vi "Threshold and Subsample Image.vi"(6 "Subsample":i32=1, 9 "Threshold":u8, 10 "Direction to keep":enum16{"Above", "Below"}(ring), 11 "Image Pixels (U8)":u8[][](array[numeric])) -> (1 "Cross Threshold Points":cluster{"X":i32, "Y":i32}[](array[cluster]), 3 "Image Pixels (U8) out":u8[][](array[numeric]))   [LabVIEW 2013]
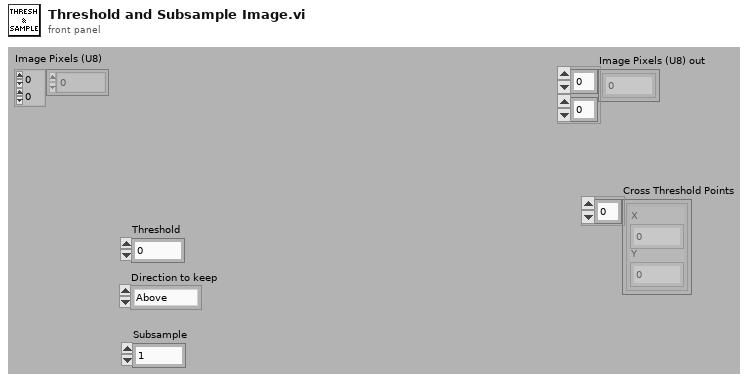
[diagram p1: front panel]
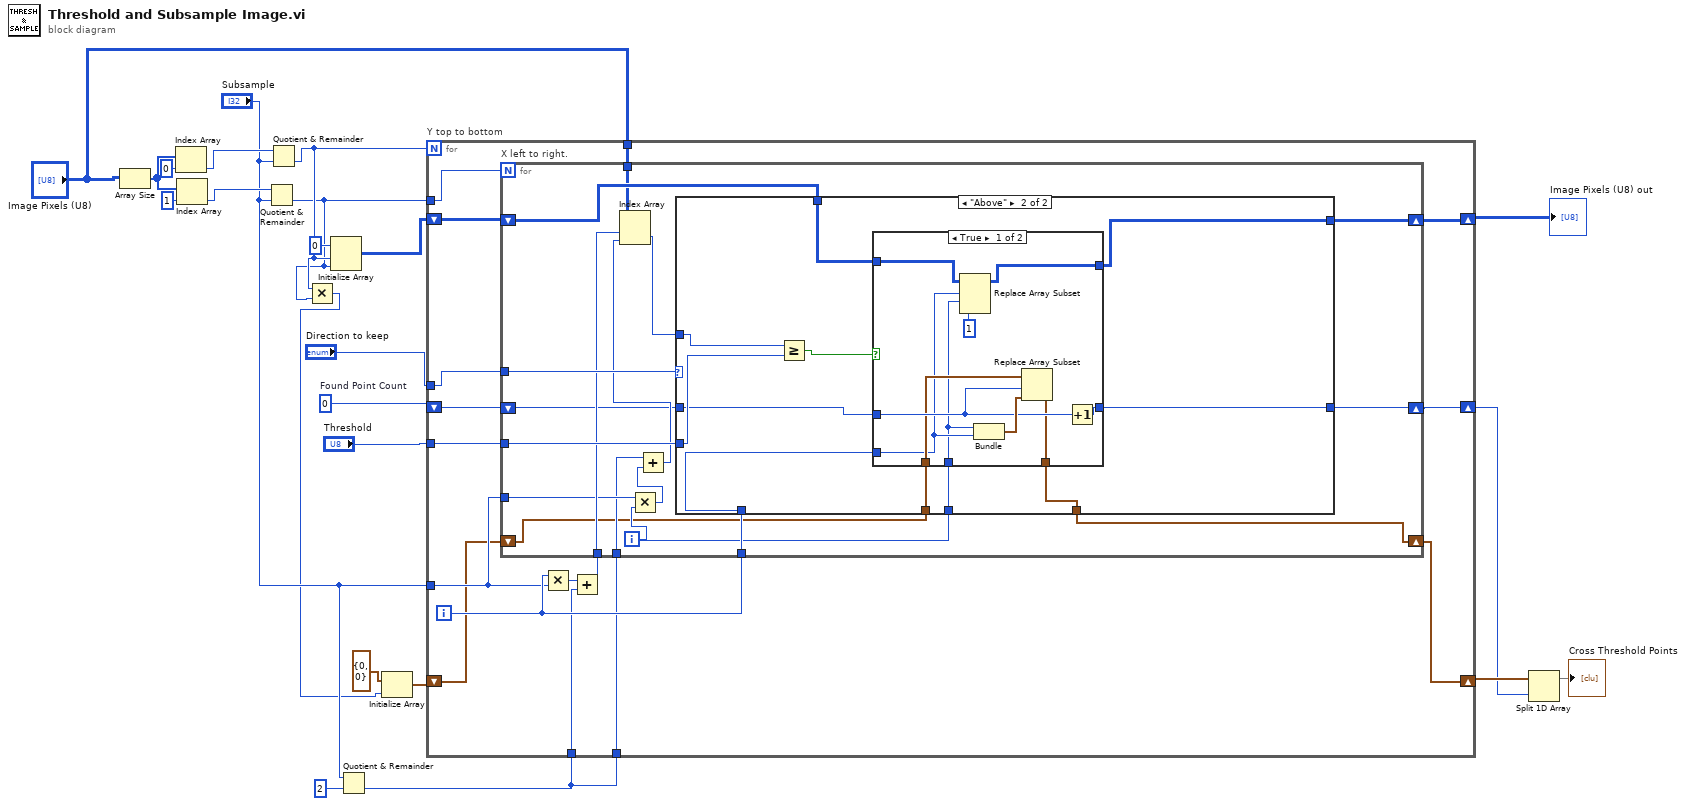
[diagram p0: block diagram]
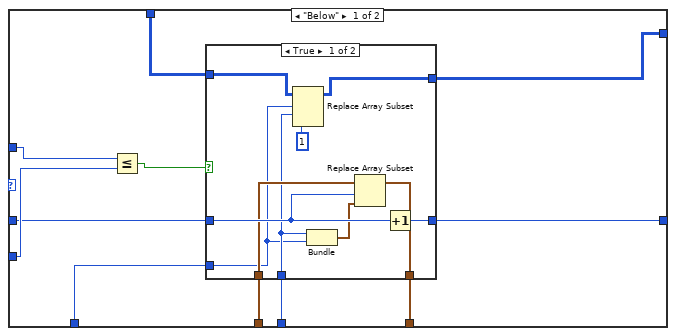
[diagram p2: hidden frame]
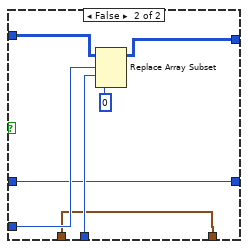
[diagram p3: hidden frame]
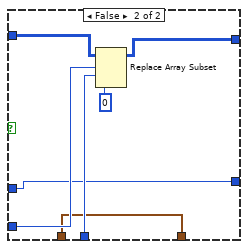
[diagram p4: hidden frame]
diagram:
  w9 = 0  # Found Point Count
  n1 = Array Size(array="Image Pixels (U8)") -> (size(s)=w20:i32[])
  n2 = Index Array(array=w20, index=0) -> (element=w17:i32)
  n3 = Index Array(array=w20, index=1) -> (element=w16:i32)
  n4 = Quotient & Remainder(x=w16, y="Subsample") -> (floor(x/y)=w6:i32)  [unwired: 1 out]
  n5 = Quotient & Remainder(x=w17, y="Subsample") -> (floor(x/y)=w7:i32)  [unwired: 1 out]
  n6 = Multiply(x=w7, y=w6) -> (x*y=w5:i32)
  n7 = Initialize Array(u8 0 ("element"), w7, w6) -> (w13:u8[][])
  n8 = Quotient & Remainder(x="Subsample", y=2) -> (floor(x/y)=w10:i32)  [unwired: 1 out]
  n9 = Initialize Array(cluster{"X":i32, "Y":i32} {"X"=0, "Y"=0} ("Point Coordinates"), w5) -> (w4:cluster{"X":i32, "Y":i32}[])
  n10 = for "Y top to bottom" {
    N: w7 -> [_]
    tunnel: "Direction to keep" -> [w39]
    tunnel: "Threshold" -> [w38]
    shift-right: [w36] -> w23
    shift-left: w13 -> [w37]
    tunnel: w6 -> [w35]
    tunnel: "Subsample" -> [w33]
    tunnel: "Image Pixels (U8)" -> [w32]
    tunnel: w10 -> [w30]
    tunnel: w10 -> [w28]
    shift-right: [w26] -> w2
    shift-left: w9 -> [w27]
    shift-right: [w24] -> w3
    shift-left: w4 -> [w25]
    i -> [w34]
    n11 = Multiply(x=w34, y=w33) -> (x*y=w31:i32)
    n12 = Add(x=w31, y=w30) -> (x+y=w29:i32)
    n13 = for "X left to right." {
      N: w35 -> [_]
      tunnel: w29 -> [w52]
      tunnel: w39 -> [w56]
      tunnel: w38 -> [w54]
      shift-right: [w53] -> w36
      shift-left: w37 -> [w48]
      tunnel: w34 -> [w51]
      tunnel: w33 -> [w49]
      tunnel: w32 -> [w47]
      tunnel: w28 -> [w44]
      shift-right: [w42] -> w26
      shift-left: w27 -> [w43]
      shift-right: [w40] -> w24
      shift-left: w25 -> [w41]
      i -> [w50]
      n14 = Multiply(x=w49, y=w50) -> (x*y=w46:i32)
      n15 = Add(x=w44, y=w46) -> (x+y=w45:i32)
      n16 = Index Array(array=w47, index (row)=w52, index (col)=w45) -> (element=w55:u8)
      n17 = case shown="\"Above\"" w56 {
        tunnel: w55 -> [w61 w89]
        tunnel: w54 -> [w67 w95]
        tunnel: w48 -> [w65 w93]
        tunnel: [w64 w92] -> w53
        tunnel: w51 -> [w63 w91]
        tunnel: w50 -> [w62 w90]
        tunnel: w43 -> [w60 w88]
        tunnel: [w59 w87] -> w42
        tunnel: w41 -> [w58 w86]
        tunnel: [w57 w85] -> w40
        frame "Below" {
          n18 = Less Or Equal?(x=w61, y=w67) -> (x <= y?=w66:bool)
          n19 = case shown="True" w66 {
            tunnel: w65 -> [w77 w84]
            tunnel: [w75 w80] -> w64
            tunnel: w63 -> [w69 w83]
            tunnel: w62 -> [w70 w82]
            tunnel: w60 -> [w73 w79]
            tunnel: [w74 w79] -> w59
            tunnel: w58 -> [w72 w78]
            tunnel: [w71 w78] -> w57
            frame True {
              n20 = Replace Array Subset(array=w77, new element=u8 1 ("new element/subarray"), index (row)=w69, index (col)=w70) -> (w75:u8[][])
              n21 = Bundle(w70, w69) -> (w68:cluster{i32, i32})  [unwired: 1 in]
              n22 = Replace Array Subset(array=w72, new element=w68, index=w73) -> (w71:cluster{"X":i32, "Y":i32}[])
              n23 = Increment(x=w73) -> (x+1=w74:i32)
            }
            frame False {
              n24 = Replace Array Subset(array=w84, new element=u8 0 ("new element/subarray"), index (row)=w83, index (col)=w82) -> (w80:u8[][])
            }
          }
        }
        frame "Above" {
          n25 = Greater Or Equal?(x=w89, y=w95) -> (x >= y?=w94:bool)
          n26 = case shown="True" w94 {
            tunnel: w93 -> [w105 w112]
            tunnel: [w103 w108] -> w92
            tunnel: w91 -> [w97 w111]
            tunnel: w90 -> [w96 w110]
            tunnel: w88 -> [w100 w107]
            tunnel: [w102 w107] -> w87
            tunnel: w86 -> [w99 w106]
            tunnel: [w98 w106] -> w85
            frame True {
              n27 = Replace Array Subset(array=w105, new element=u8 1 ("new element/subarray"), index (row)=w97, index (col)=w96) -> (w103:u8[][])
              n28 = Bundle(w96, w97) -> (w101:cluster{i32, i32})  [unwired: 1 in]
              n29 = Replace Array Subset(array=w99, new element=w101, index=w100) -> (w98:cluster{"X":i32, "Y":i32}[])
              n30 = Increment(x=w100) -> (x+1=w102:i32)
            }
            frame False {
              n31 = Replace Array Subset(array=w112, new element=u8 0 ("new element/subarray"), index (row)=w111, index (col)=w110) -> (w108:u8[][])
            }
          }
        }
      }
    }
  }
  "Image Pixels (U8) out" <- w23
  n32 = Split 1D Array(array=w3, index=w2) -> (first subarray=→"Cross Threshold Points":cluster{"X":i32, "Y":i32}[])  [unwired: 1 out]
